vi "GetCloserEnd.vi"(1 "Destination":cluster{"x":dbl, "y":dbl}, 2 "Robot Pos":cluster{"x":dbl, "y":dbl, "angle":dbl}) -> (0 "Forward Closer":bool)   [LabVIEW 2015, in "Navigation2017.lvlib" / "Navigation2017-SubVIs.lvlib"]
doc: "Given a robot position and spin, figures out which end of the robot is closest to a destination x and y. Returns true for front, and false for back.\n\nFirst written William Karnavas, Spring 2017"
uses:
  Navigation2017-SubVIs.lvlib
  Navigation2017-util.lvlib
panel:
  # "Returns:\nTrue - Front Closer\nFalse - Back Closer"
  # "Given a robot position and spin, figures out which end of the robot is closest to a destination x and y. Returns 1 for front, and 2 for back.\n\nFirst written William Karnavas, Spr 2017"
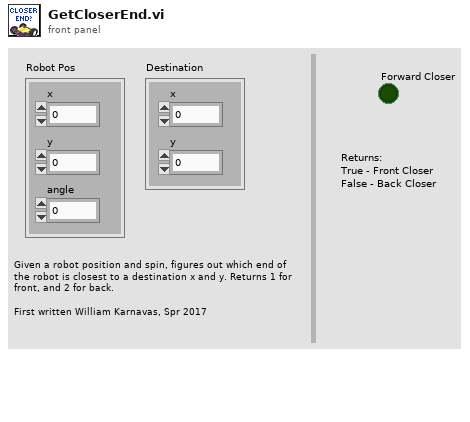
[diagram p1: front panel]
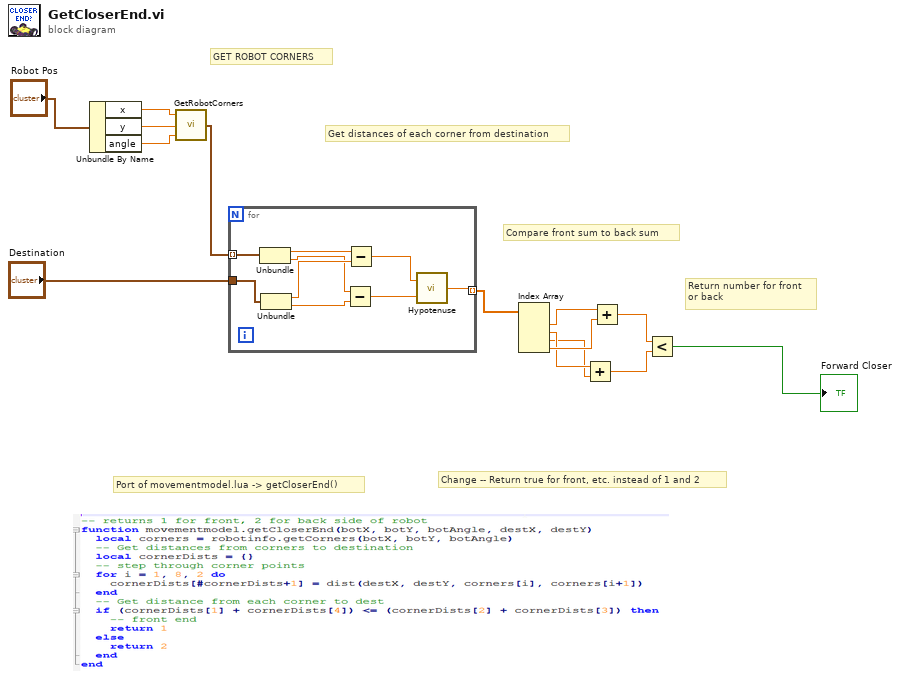
[diagram p0: block diagram]
diagram:
  # "Change -- Return true for front, etc. instead of 1 and 2"
  # "Port of movementmodel.lua -> getCloserEnd()"
  # "Return number for front\nor back"
  # "Compare front sum to back sum"
  # "Get distances of each corner from destination"
  # "GET ROBOT CORNERS"
  n1 = Unbundle By Name("Robot Pos") -> ("x"=w13:dbl, "y"=w12:dbl, "angle"=w11:dbl)
  n2 = call "GetRobotCorners.vi"("botAngle (rad)"=w11, "botY (m)"=w12, "botX (m)"=w13) -> ("Corner Points (m)"=w9:cluster{dbl, dbl}[])
  n3 = for {
    tunnel: [w23] -> w10 mode=indexing
    tunnel: w9 -> [w22] mode=indexing
    tunnel: "Destination" -> [w21]
    n4 = Unbundle(w22) -> (w20:dbl, w17:dbl)
    n5 = Unbundle(w21) -> ("x"=w19:dbl, "y"=w16:dbl)
    n6 = Subtract(x=w17, y=w16) -> (x-y=w15:dbl)
    n7 = Subtract(x=w20, y=w19) -> (x-y=w18:dbl)
    n8 = call "Hypotenuse.vi"("y"=w15, "x"=w18) -> ("r"=w23:dbl)
  }
  n9 = Index Array(array=w10) -> (element #1=w7:dbl, element #2=w5:dbl, element #3=w4:dbl, element #4=w6:dbl)  [unwired: 4 in]
  n10 = Add(x=w5, y=w4) -> (x+y=w2:dbl)
  n11 = Add(x=w7, y=w6) -> (x+y=w3:dbl)
  n12 = Less?(x=w3, y=w2) -> (x < y?=→"Forward Closer":bool)
